vi "Tester.vi"   [LabVIEW 2016, in "Event Actors.lvlib" / "Controller Actor.lvclass"]
uses:
  Controller Actor.lvclass
  Event/Event.lvclass
  Event Handlers/Event Generated Msg/Event Generated Msg.lvclass
  <vilib>/ActorFramework/Message Queue/Message Queue.lvclass
  <vilib>/ActorFramework/Message Dequeuer/Message Dequeuer.lvclass
  <vilib>/ActorFramework/Message Enqueuer/Message Enqueuer.lvclass
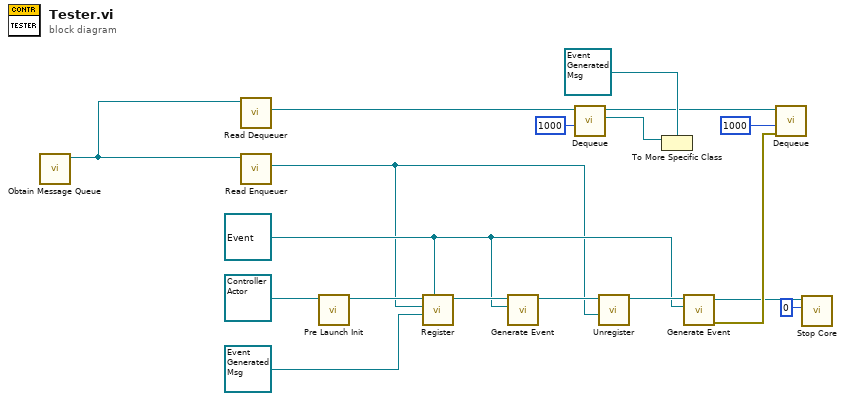
[diagram p0: block diagram]
diagram:
  w3 = refnum<class "Event.lvclass"> refnum ("Event Source.lvlib:Event.lvclass")
  n1 = call <vilib>:"Obtain Message Queue.vi"() -> ("Message Queue"=w18:refnum<class "Message Queue.lvclass">)  [unwired: 10 in, 1 out]
  n2 = call <vilib>:"Read Dequeuer.vi"("Message Queue"=w18) -> ("Message Dequeuer"=w17:refnum<class "Message Dequeuer.lvclass">)  [unwired: 10 in]
  n3 = call <vilib>:"Read Enqueuer.vi"("Message Queue"=w18) -> ("Message Enqueuer"=w2:refnum<class "Message Enqueuer.lvclass">)  [unwired: 10 in]
  n4 = call-dynamic "Pre Launch Init.vi"("Event Source In"=refnum<class "Controller Actor.lvclass"> refnum ("Event Source.lvlib:Event Source.lvclass")) -> ("Event Source Out"=w5:refnum<class "Controller Actor.lvclass">)  [unwired: 9 in, 1 out]
  n5 = call "Register.vi"("Event"=w3, "Sink Event Fire Handler"=refnum<class "Event Generated Msg.lvclass"> refnum ("Event Source.lvlib:Event Fired Msg.lvclass"), "Registrant Details"=w2, "Event Source In"=w5) -> ("Event Source Out"=w6:refnum<class "Controller Actor.lvclass">)  [unwired: 6 in, 1 out]
  n6 = call "Generate Event.vi"("Event"=w3, "Event Source In"=w6) -> ("Event Source Out"=w4:refnum<class "Controller Actor.lvclass">)  [unwired: 8 in, 1 out]
  n7 = call <vilib>:"Dequeue.vi"("timeout in ms (-1)"=1000, "Message Dequeuer in"=w17) -> ("Message"=w16:refnum<class "Message.lvclass">, "Message Dequeuer out"=w13:refnum<class "Message Dequeuer.lvclass">)  [unwired: 5 in, 3 out]
  n8 = call "Unregister.vi"("Registrant Enq"=w2, "Event Source In"=w4) -> ("Event Source Out"=w14:refnum<class "Controller Actor.lvclass">)  [unwired: 8 in, 1 out]
  n9 = To More Specific Class(target class=refnum<class "Event Generated Msg.lvclass"> refnum ("Event Source.lvlib:Event Fired Msg.lvclass"), reference=w16) -> ()  [unwired: 1 in, 2 out]
  n10 = call "Generate Event.vi"("Event"=w3, "Event Source In"=w14) -> ("Error Out"=w11:errorcluster, "Event Source Out"=w9:refnum<class "Controller Actor.lvclass">)  [unwired: 8 in]
  n11 = call <vilib>:"Dequeue.vi"("error in (no error)"=w11, "timeout in ms (-1)"=1000, "Message Dequeuer in"=w13) -> ()  [unwired: 4 in, 5 out]
  n12 = call-dynamic "Stop Core.vi"("final error code"=0, "Event Source In"=w9) -> ()  [unwired: 9 in, 1 out]
